vi "Add New Waveform Channel.vi"(0 "Node Ptr":T1 format="%.0x") -> ()   [LabVIEW 2023, in "Embedded TDMS Logger System Explorer.lvlib"]
uses:
  Embedded TDMS Logger System Explorer.lvlib
  <vilib>/NI VeriStand/Custom Device API/Custom Device Item Ref.ctl
  Shared/Meta Data Item.ctl
  Shared/Constants.vi
  <vilib>/NI VeriStand/Custom Device API/Set Item Property (Boolean).vi
  <vilib>/NI VeriStand/Custom Device API/Set Item Property (Dependent Node Pointer).vi
  <vilib>/NI VeriStand/Custom Device API/Set Item Property (Variant).vi
  Shared/Embedded TDMS Logger Shared.lvlib
  <vilib>/NI VeriStand/Custom Device API/Custom Device API.lvlib
  <vilib>/NI VeriStand/Custom Device Tools/Custom Device Utility Library/Custom Device Utility Library.lvlib
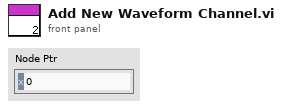
[diagram p1: front panel]
types:
  T1 = typedef "Custom Device API.lvlib/Custom Device Item Ref.ctl" = u64
  T2 = typedef "Embedded TDMS Logger Shared.lvlib/Meta Data Item.ctl" = cluster{"Key":string, "Value":string}
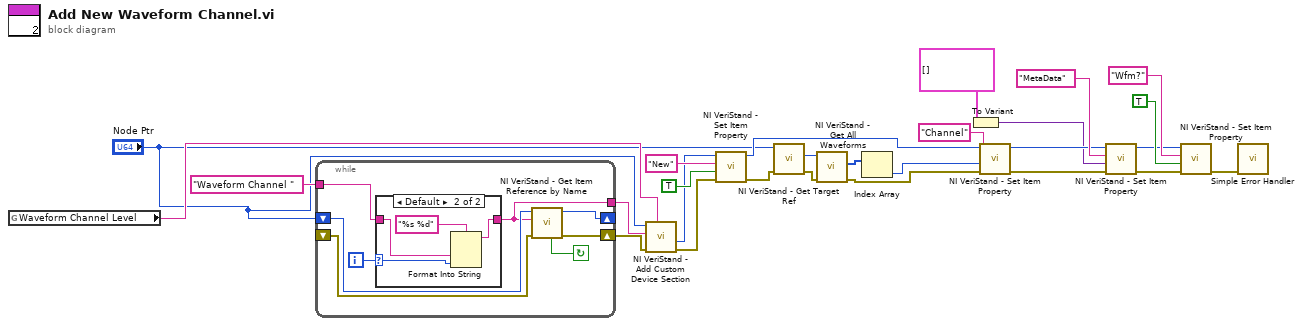
[diagram p0: block diagram]
diagram:
  n1 = global read "Constants.vi" "Waveform Channel Level"() -> (w27:string)
  n2 = while {
    shift-right: [w29] -> w24
    shift-left: _ -> [w33]
    shift-right: [w31] -> _
    shift-left: "Node Ptr" -> [w32]
    tunnel: "Waveform Channel " ("group name") -> [w34]
    tunnel: [w28] -> w25
    i -> [w35]
    stop <- w30 continue-if-true
    n3 = case shown="Default" w35 {
      selector: w35 -> [_ w38]
      tunnel: w34 -> [w36 w39]
      tunnel: [w36 w37] -> w28
      frame 0 {
      }
      frame Default {
        n4 = Format Into String(format string="%s %d", w39, w38) -> (resulting string=w37:string)  [unwired: 2 in, 1 out]
      }
    }
    n5 = call <vilib>:"NI VeriStand - Get Item Reference by Name.vi"("error in (no error)"=w33, "Item Name"=w28, "Parent Ref in"=w32) -> ("error out"=w29:errorcluster, "Parent Ref out"=w31:T1, "Found"=w30:bool)  [unwired: 6 out]
  }
  n6 = call <vilib>:"NI VeriStand - Add Custom Device Section.vi"("GUID (Default Section)"=w27, "error in (no error)"=w24, "Section Name"=w25, "Parent Ref in"="Node Ptr") -> ("error out"=w21:errorcluster, "Section Ptr"=w20:T1)  [unwired: 3 in, 3 out]
  n7 = call-poly <vilib>:"NI VeriStand - Set Item Property.vi"("error in (no error)"=w21, "Value"=TRUE, "Property Name"="New", "Item Ref in"=w20) -> ("error out"=w14:errorcluster, "Item Ref out"=w2:T1)  [unwired: 5 in, 1 out]
  n8 = call <vilib>:"NI VeriStand - Get Target Ref.vi"("error in"=w14, "Item Ref in"="Node Ptr") -> ("error out"=w16:errorcluster, "Target Ref"=w15:T1)  [unwired: 6 in, 2 out]
  n9 = call <vilib>:"NI VeriStand - Get All Waveforms.vi"("error in"=w16, "Section Ref in"=w15) -> ("error out"=w11:errorcluster, "Waveform Refs"=w13:T1[])  [unwired: 6 in, 2 out]
  n10 = Index Array(array=w13) -> (element=w12:T1)  [unwired: 1 in]
  n11 = To Variant(anything=T2[] []) -> (Variant=w5:variant)
  n12 = call-poly <vilib>:"NI VeriStand - Set Item Property.vi"("error in (no error)"=w11, "Dependent Node Ref"=w12, "Property Name"="Channel", "Item Ref in"=w2) -> ("error out"=w9:errorcluster, "Item Ref out"=w8:T1)  [unwired: 5 in, 1 out]
  n13 = call-poly <vilib>:"NI VeriStand - Set Item Property.vi"("error in (no error)"=w9, "Value"=w5, "Property Name"="MetaData", "Item Ref in"=w8) -> ("error out"=w6:errorcluster, "Item Ref out"=w7:T1)  [unwired: 5 in, 1 out]
  n14 = call-poly <vilib>:"NI VeriStand - Set Item Property.vi"("error in (no error)"=w6, "Value"=TRUE, "Property Name"="Wfm?", "Item Ref in"=w7) -> ("error out"=w17:errorcluster)  [unwired: 5 in, 2 out]
  n15 = call <vilib>:"Simple Error Handler.vi"("error in (no error)"=w17) -> ()  [unwired: 4 in, 5 out]
